vi "set Temperature LV.vi"(8 "error in (no error)":errorcluster, 11 "setTemp":i32) -> (0 "error out":errorcluster)   [LabVIEW 2016, in "cameraLibrary.lvlib"]
doc: "Set the target array temperature.\n\n\nvoid CAMERALIBRARYSHARED_EXPORT setTemperatureLV(int setTemp);"
uses:
  cameraLibrary.lvlib
  cameraLibrary.dll
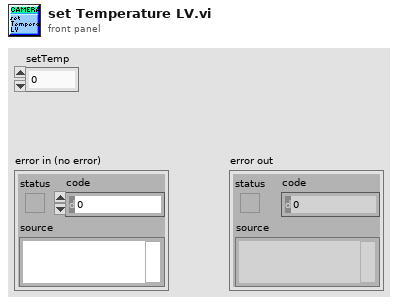
[diagram p1: front panel]
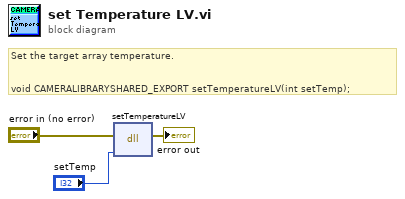
[diagram p0: block diagram]
diagram:
  # "Set the target array temperature.\n\n\nvoid CAMERALIBRARYSHARED_EXPORT setTemperatureLV(int setTemp);"
  n1 = dll-call lib="C:/Users/TMM/repos/EXPRES/FEM/FTT/support/Camera Library/cameraLibrary.*" fn="setTemperatureLV"(error in="error in (no error)", "setTemp"="setTemp") -> (error out=→"error out":errorcluster)  [unwired: 4 in, 1 out]
